vi "hamamatsu error parse.vi"(11 "return type":u16) -> (0 "error out":errorcluster)   [LabVIEW 2013]
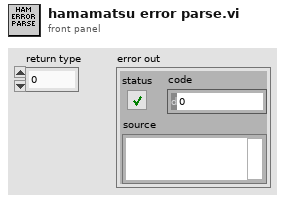
[diagram p1: front panel]
types:
  T1 = typedef "specu1a 1.0.0 Error codes.ctl" = enum16{"INVALID_HANDLE_VALUE", "USBDEV_SUCCESS", "USBDEV_INVALID_HANDLE", "USBDEV_UNSUCCESS", "USBDEV_INVALID_VALUE", "USBDEV_CHECK_NORMAL", "USBDEV_CHECK_INVALID", "USBDEV_CHECK_REMOVE", "USBDEV_CHECK_OTHER", "USBDEV_RESET_ERROR", "USBDEV_BULKSIZE_ERROR", "USBDEV_BULK_READ_ERROR", "USBDEV_BULK_NOT_UPDATED", "USBDEV_TIME_OVER_ERROR", "USBDEV_TIME_UNDER_ERROR", "USBDEV_TIME_SET_ERROR", "USBDEV_SET_GAIN_ERROR", "USBDEV_GET_TEMP_ERROR", "USBDEV_SET_TRIGGER_ERROR", "USBDEV_RW_EEP_ADDR_ERROR", "USBDEV_RW_EEP_SIZE_ERROR", "USBDEV_RW_EEP_OVER_ERROR", "USBDEV_RW_EEP_ERROR", "UNITID_PRODUCTID_CONFLICT", "UNKNOWN_ERROR"}
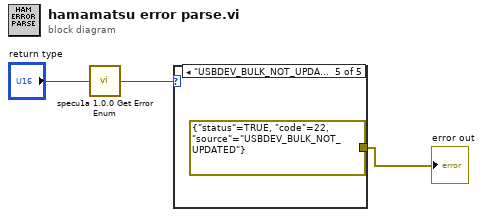
[diagram p0: block diagram]
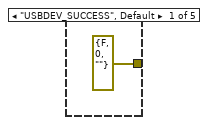
[diagram p2: hidden frame]
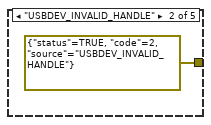
[diagram p3: hidden frame]
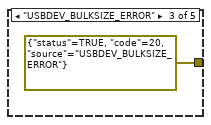
[diagram p4: hidden frame]
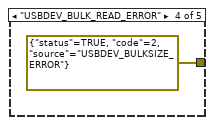
[diagram p5: hidden frame]
diagram:
  n1 = call "specu1a 1.0.0 Get Error Enum.vi"("Error Code in"="return type") -> ("Specu1a 1.0.0 Error code out"=w3:T1)  [unwired: 4 in]
  n2 = case shown="\"USBDEV_BULK_NOT_UPDATED\"" w3 {
    tunnel: [errorcluster {"status"=FALSE, "code"=0, "source"=""} ("error out") errorcluster {"status"=TRUE, "code"=2, "source"="USBDEV_INVALID_HANDLE"} ("error out") errorcluster {"status"=TRUE, "code"=20, "source"="USBDEV_BULKSIZE_ERROR"} ("error out") errorcluster {"status"=TRUE, "code"=2, "source"="USBDEV_BULKSIZE_ERROR"} ("error out") errorcluster {"status"=TRUE, "code"=22, "source"="USBDEV_BULK_NOT_UPDATED"} ("error out")] -> w1
    frame "USBDEV_SUCCESS", Default {
    }
    frame "USBDEV_INVALID_HANDLE" {
    }
    frame "USBDEV_BULKSIZE_ERROR" {
    }
    frame "USBDEV_BULK_READ_ERROR" {
    }
    frame "USBDEV_BULK_NOT_UPDATED" {
    }
  }
  "error out" <- w1
